vi "Write Config.vi"(8 "error in (no error)":errorcluster, 10 "Config":T1={"Folder Pattern"="%s:\\", "Starting Letter Position"=3, "Min Free Space (MB)"=50.0, "Max Folders to Check"=10, "Trace Level"=enum."Informational"} {"Min Free Space (MB)" format="%#_13g"}, 11 "Trace Controller in":refnum<class "Trace Controller.lvclass">) -> (0 "error out":errorcluster, 3 "Trace Controller out":refnum<class "Trace Controller.lvclass">)   [LabVIEW 2014, in "Robot Actor Framework.lvlib" / "Trace.lvlib" / "Trace Controller.lvclass"]
uses:
  Trace Controller.lvclass
  Config.ctl
  Trace Controller.lvclass/Trace Controller.ctl
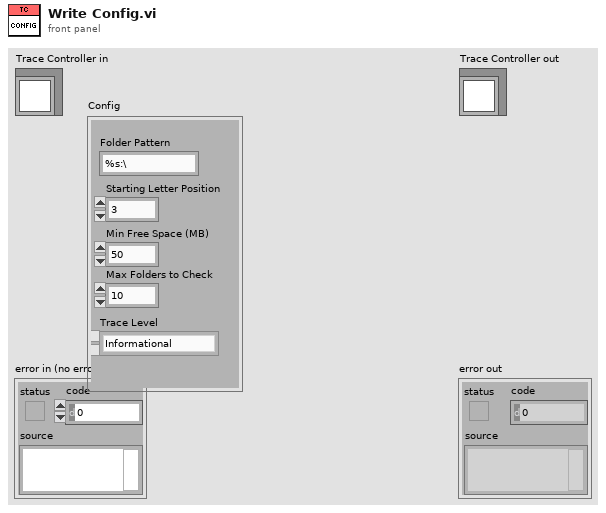
[diagram p1: front panel]
types:
  T1 = typedef "Robot Actor Framework.lvlib/Trace.lvlib/Trace Controller.lvclass/Config.ctl" = cluster{"Folder Pattern":string, "Starting Letter Position":i32, "Min Free Space (MB)":dbl, "Max Folders to Check":u32, "Trace Level":enum16{"Critical", "Error", "Warning", "Informational", "Debug"}}
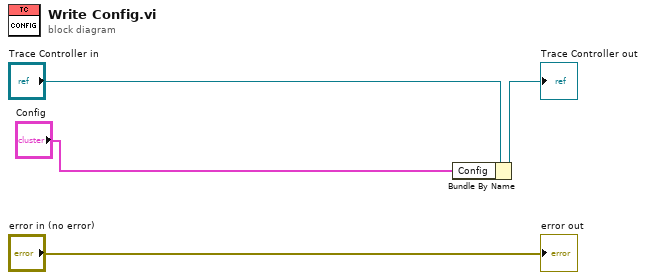
[diagram p0: block diagram]
diagram:
  n1 = Bundle By Name(cluster="Trace Controller in", "Config"="Config") -> (→"Trace Controller out":refnum<class "Trace Controller.lvclass">)
  "error out" <- "error in (no error)"
